vi "InputPad.vi"() -> (3 "PadIndicator":dbl format="%6.2f")   [LabVIEW 2012, in "StimulCtrls.lvlib"]
uses:
  StimulCtrls.lvlib
  PadEnum.ctl
panel:
  in  "Enter":bool
  in  "Backspace":bool
  in  "Clear":bool
  in  "Up":bool
  in  "Down":bool
  in  "Dot":bool
  in  "NUM 9":bool
  in  "NUM 8":bool
  in  "NUM 7":bool
  in  "NUM 6":bool
  in  "NUM 5":bool
  in  "NUM 4":bool
  in  "NUM 3":bool
  in  "NUM 2":bool
  in  "NUM 1":bool
  in  "NUM 0":bool
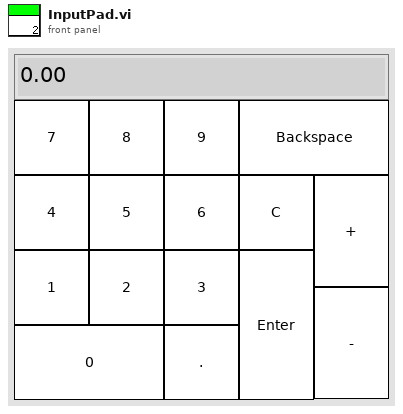
[diagram p1: front panel]
types:
  T1 = typedef "PadEnum.ctl" = enum16{"Clear", "Increase", "Decrease", "Wait", "Exit", "Backspace", "InputDigit"}
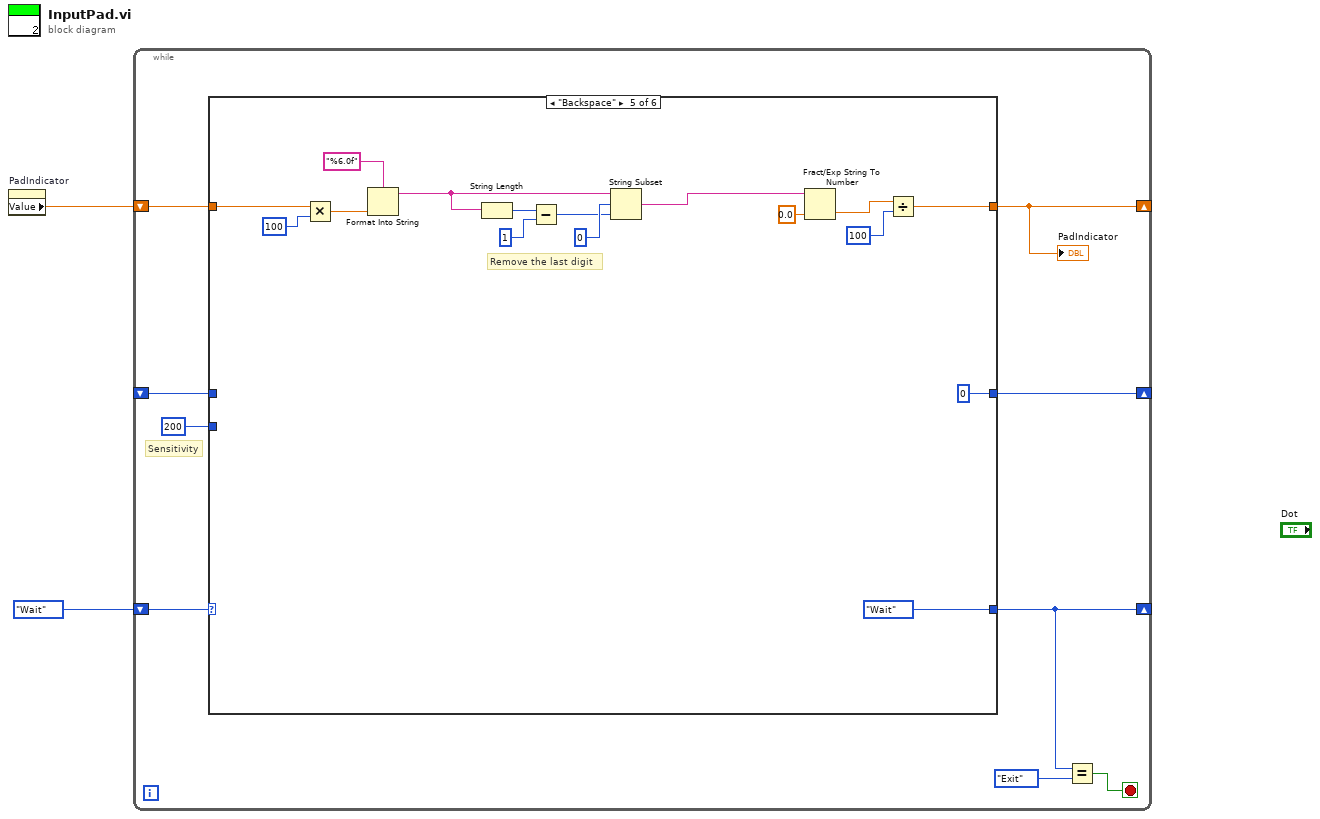
[diagram p0: block diagram]
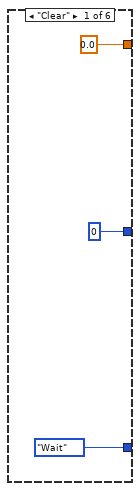
[diagram p2: hidden frame]
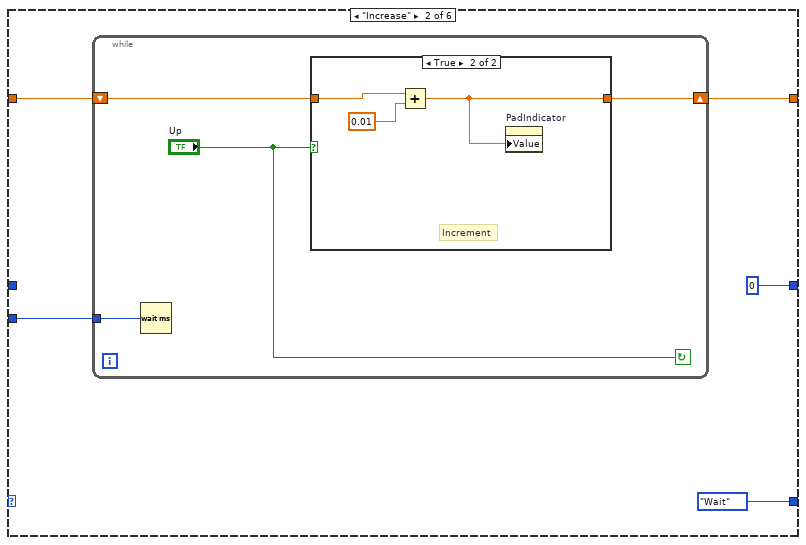
[diagram p3: hidden frame]
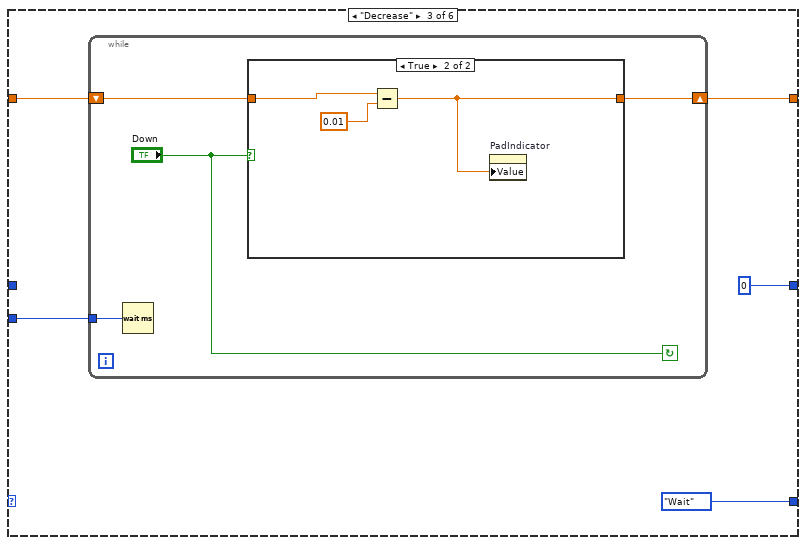
[diagram p5: hidden frame]
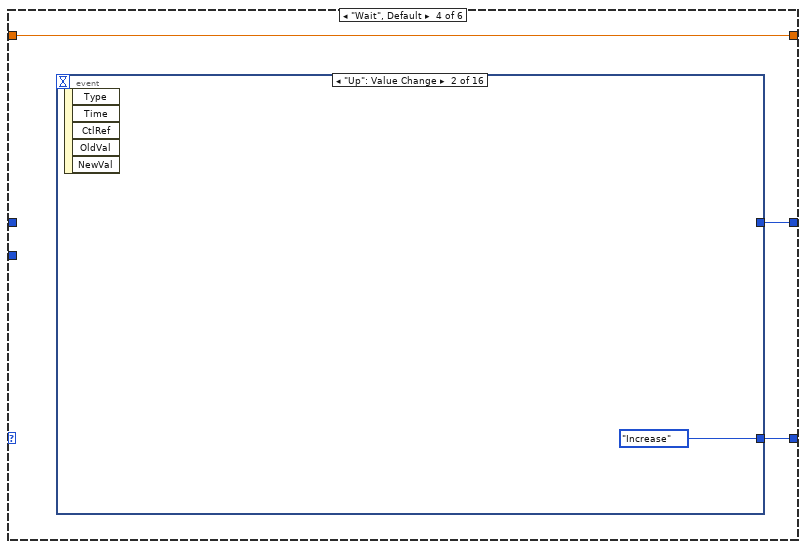
[diagram p7: hidden frame]
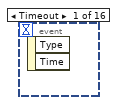
[diagram p8: hidden frame]
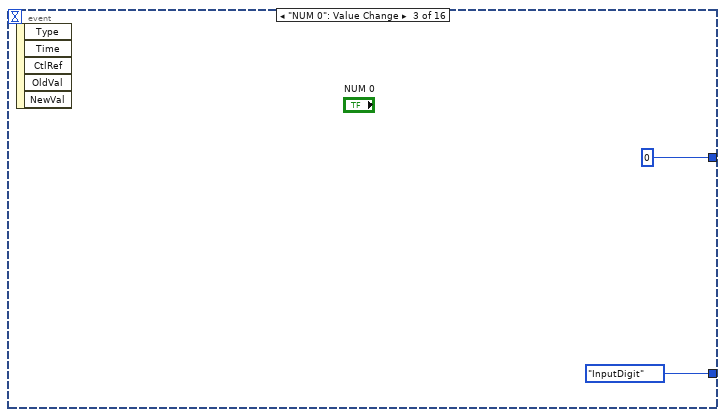
[diagram p9: hidden frame]
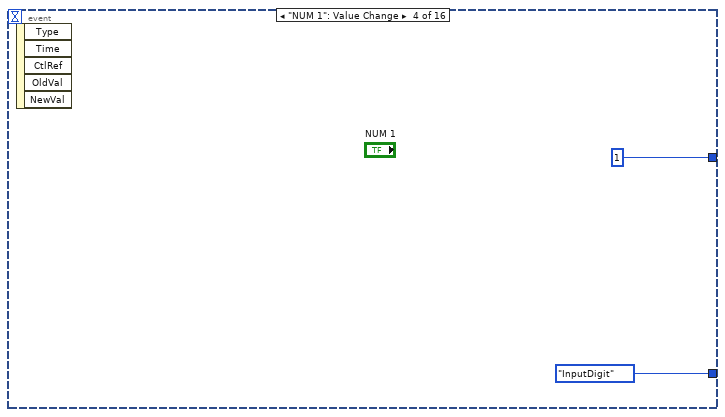
[diagram p10: hidden frame]
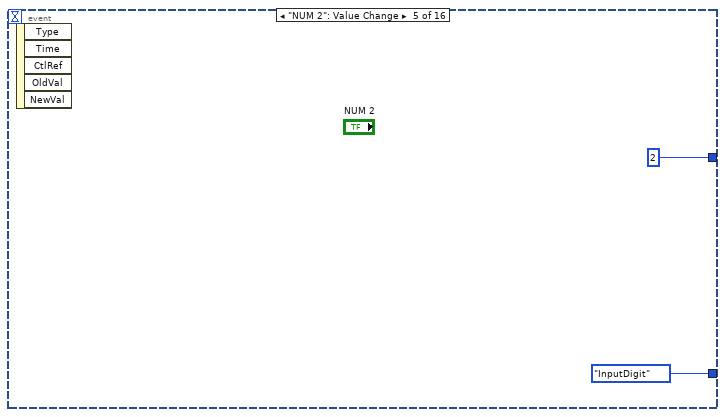
[diagram p11: hidden frame]
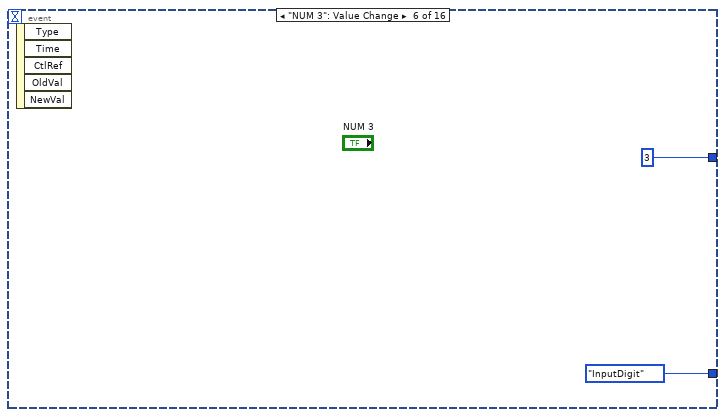
[diagram p12: hidden frame]
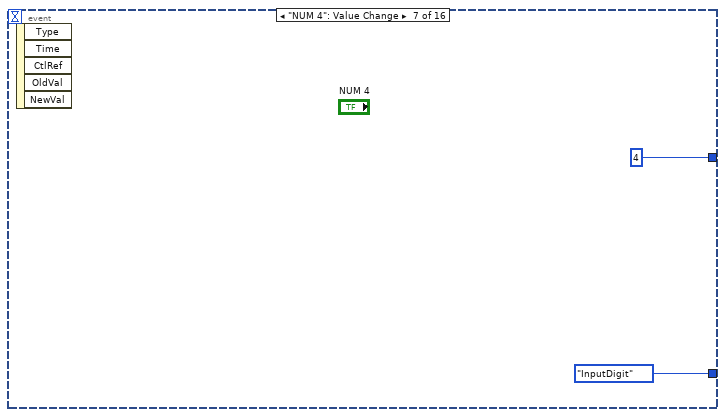
[diagram p13: hidden frame]
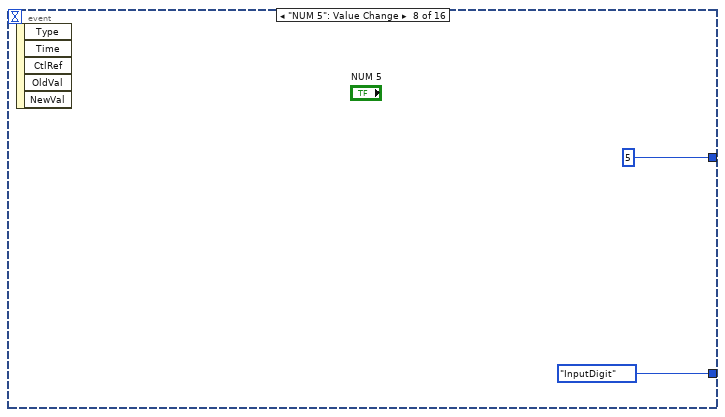
[diagram p14: hidden frame]
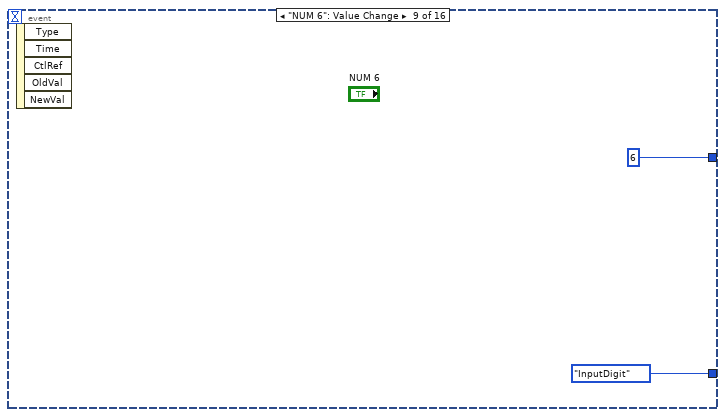
[diagram p15: hidden frame]
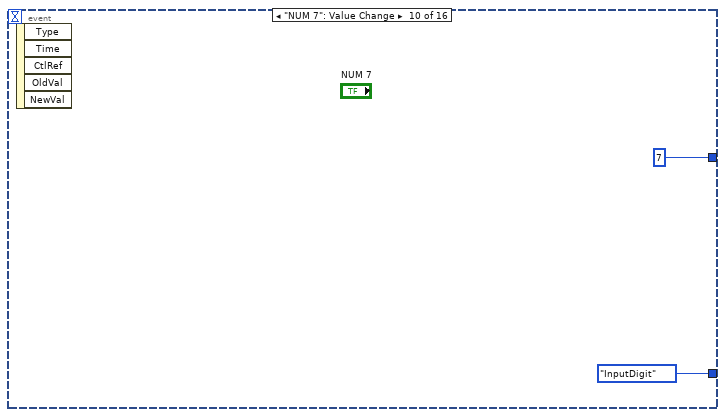
[diagram p16: hidden frame]
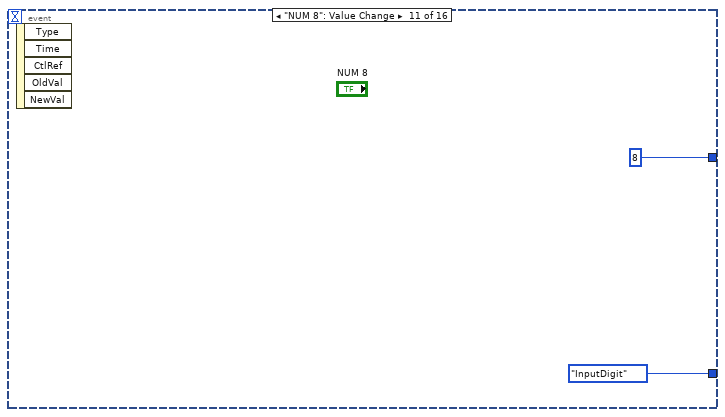
[diagram p17: hidden frame]
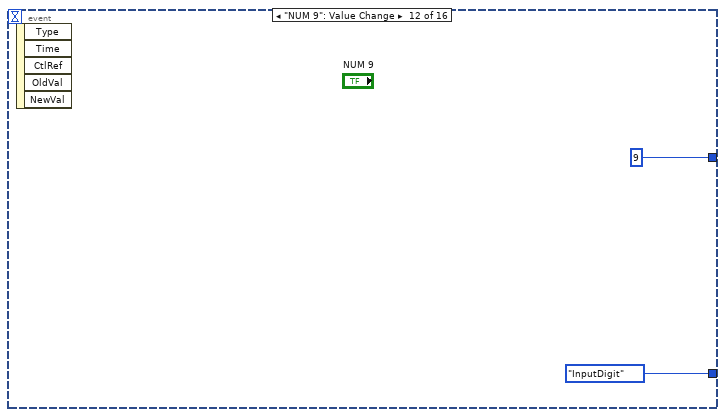
[diagram p18: hidden frame]
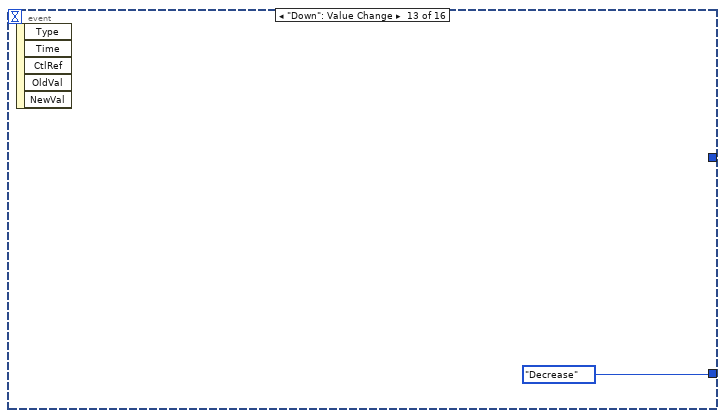
[diagram p19: hidden frame]
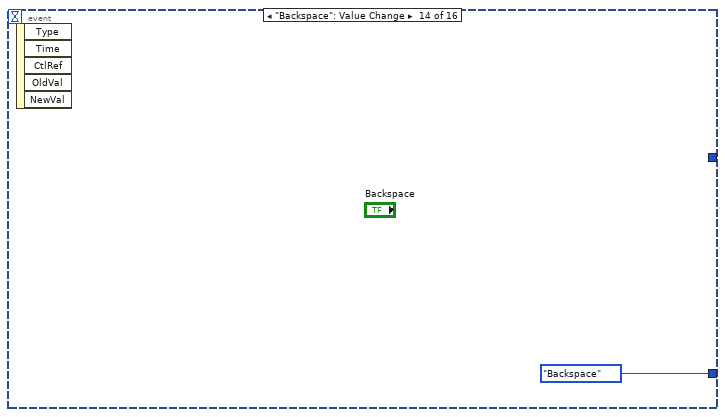
[diagram p20: hidden frame]
diagram:
  n1 = property on="PadIndicator" class="DigNum (strict)"() -> ("Value"=w1:dbl)  [unwired: 2 in, 2 out]
  n2 = while {
    shift-right: [w6] -> _
    shift-left: PadEnum."Wait" -> [w10]
    shift-right: [w8] -> _
    shift-left: w1 -> [w9]
    shift-right: [w5] -> _
    shift-left: _ -> [w4]
    stop <- w11 stop-if-true
    # "Sensitivity"
    n3 = case shown="\"Backspace\"" w10 {
      tunnel: [PadEnum."Wait" ("x") PadEnum."Wait" ("x") PadEnum."Wait" ("x") w43 PadEnum."Wait" ("x") PadEnum."Wait" ("x")] -> w6
      tunnel: [0.0 w18 w31 w42 w77 w85] -> w8
      tunnel: w9 -> [_ w19 w32 w42 w82 w96]
      tunnel: [0 0 0 w41 0 0] -> w5
      tunnel: w4 -> [_ _ _ _ _ w92]
      tunnel: u32 200 ("milliseconds to wait") -> [_ w15 w28 _ _ _]
      frame "Clear" {
      }
      frame "Increase" {
        n4 = while {
          shift-right: [w22] -> w18
          shift-left: w19 -> [w23]
          tunnel: w15 -> [w21]
          stop <- "Up" continue-if-true
          n5 = Wait (ms)(milliseconds to wait=w21) -> ()  [unwired: 1 out]
          n6 = case shown="True" "Up" {
            tunnel: w23 -> [w24 w26]
            tunnel: [w24 w25] -> w22
            frame False {
            }
            frame True {
              # "Increment"
              n7 = Add(x=w26, y=0.01) -> (x+y=w25:dbl)
              n8 = property on="PadIndicator" class="DigNum (strict)"("Value"=w25) -> ()  [unwired: 2 in, 2 out]
            }
          }
        }
      }
      frame "Decrease" {
        n9 = while {
          shift-right: [w35] -> w31
          shift-left: w32 -> [w36]
          tunnel: w28 -> [w34]
          stop <- "Down" continue-if-true
          n10 = Wait (ms)(milliseconds to wait=w34) -> ()  [unwired: 1 out]
          n11 = case shown="True" "Down" {
            tunnel: w36 -> [w37 w39]
            tunnel: [w37 w38] -> w35
            frame False {
            }
            frame True {
              n12 = Subtract(x=w39, y=0.01) -> (x-y=w38:dbl)
              n13 = property on="PadIndicator" class="DigNum (strict)"("Value"=w38) -> ()  [unwired: 2 in, 2 out]
            }
          }
        }
      }
      frame "Wait", Default {
        n14 = event shown="[1] \"Up\": Value Change" {
          selector: _ -> [_ _ _ _ _ _ _ _ _ _ _ _ _ _ _ _]
          dyn-events: _ -> [_ _ _ _ _ _ _ _ _ _ _ _ _ _ _ _]
          timeout: _ -> [_ _ _ _ _ _ _ _ _ _ _ _ _ _ _ _]
          tunnel: [_ PadEnum."Increase" ("x") PadEnum."InputDigit" ("x") PadEnum."InputDigit" ("x") PadEnum."InputDigit" ("x") PadEnum."InputDigit" ("x") PadEnum."InputDigit" ("x") PadEnum."InputDigit" ("x") PadEnum."InputDigit" ("x") PadEnum."InputDigit" ("x") PadEnum."InputDigit" ("x") PadEnum."InputDigit" ("x") PadEnum."Decrease" ("x") PadEnum."Backspace" ("x") PadEnum."Clear" ("x") PadEnum."Exit" ("x")] -> w43
          tunnel: [_ _ 0 1 2 3 4 5 6 7 8 9 _ _ _ _] -> w41
          event Timeout {
            n15 = event-data() -> ()  [unwired: 1 in, 2 out]
          }
          event "Up": Value Change {
            n16 = event-data() -> ()  [unwired: 1 in, 5 out]
          }
          event "NUM 0": Value Change {
            n17 = event-data() -> ()  [unwired: 1 in, 5 out]
          }
          event "NUM 1": Value Change {
            n18 = event-data() -> ()  [unwired: 1 in, 5 out]
          }
          event "NUM 2": Value Change {
            n19 = event-data() -> ()  [unwired: 1 in, 5 out]
          }
          event "NUM 3": Value Change {
            n20 = event-data() -> ()  [unwired: 1 in, 5 out]
          }
          event "NUM 4": Value Change {
            n21 = event-data() -> ()  [unwired: 1 in, 5 out]
          }
          event "NUM 5": Value Change {
            n22 = event-data() -> ()  [unwired: 1 in, 5 out]
          }
          event "NUM 6": Value Change {
            n23 = event-data() -> ()  [unwired: 1 in, 5 out]
          }
          event "NUM 7": Value Change {
            n24 = event-data() -> ()  [unwired: 1 in, 5 out]
          }
          event "NUM 8": Value Change {
            n25 = event-data() -> ()  [unwired: 1 in, 5 out]
          }
          event "NUM 9": Value Change {
            n26 = event-data() -> ()  [unwired: 1 in, 5 out]
          }
          event "Down": Value Change {
            n27 = event-data() -> ()  [unwired: 1 in, 5 out]
          }
          event "Backspace": Value Change {
            n28 = event-data() -> ()  [unwired: 1 in, 5 out]
          }
          event "Clear": Value Change {
            n29 = event-data() -> ()  [unwired: 1 in, 5 out]
          }
          event "Enter": Value Change {
            n30 = event-data() -> ()  [unwired: 1 in, 5 out]
          }
        }
      }
      frame "Backspace" {
        # "Remove the last digit"
        n31 = Multiply(x=w82, y=100) -> (x*y=w78:dbl)
        n32 = Format Into String(format string="%6.0f", w78) -> (resulting string=w79:string)  [unwired: 2 in, 1 out]
        n33 = String Length(string=w79) -> (length=w73:i32)
        n34 = Subtract(x=w73, y=1) -> (x-y=w71:i32)
        n35 = String Subset(string=w79, offset (0)=0, length (rest)=w71) -> (substring=w81:string)
        n36 = Fract/Exp String To Number(string=w81, default (0 dbl)=0.0 ("default (0 DBL)")) -> (number=w76:dbl)  [unwired: 2 in, 1 out]
        n37 = Divide(x=w76, y=100) -> (x/y=w77:dbl)
      }
      frame "InputDigit" {
        n38 = Multiply(x=w96, y=10.0) -> (x*y=w94:dbl)
        n39 = Divide(x=w92, y=100) -> (x/y=w93:dbl)
        n40 = Add(x=w94, y=w93) -> (x+y=w86:dbl)
        n41 = Greater?(x=w86, y=1000.0) -> (0:w87:bool)
        n42 = case shown="True" w87 {
          tunnel: w86 -> [w97 w104]
          tunnel: [w97 w99] -> w85
          frame False {
          }
          frame True {
            # "Converting to \nfractional number"
            # "Removing first digit"
            # "Converting to string"
            # "To prevent the input exceeding 1000"
            n43 = Format Into String(format string="%6.2f", w104) -> (resulting string=w102:string)  [unwired: 2 in, 1 out]
            n44 = String Subset(string=w102, offset (0)=1) -> (substring=w100:string)  [unwired: 1 in]
            n45 = Scan From String(format string="%f", input string=w100) -> (output 1=w99:dbl)  [unwired: 3 in, 3 out]
          }
        }
      }
    }
    "PadIndicator" <- w8
    n46 = Equal?(x=w6, y=PadEnum."Exit" ("x")) -> (x = y?=w11:bool)
  }
